vi "Day 3 DataFlow Tasks.vi"() -> ()   [LabVIEW 2026]
panel:
  out "Final Result 7":dbl
  in  "D1 3":dbl
  in  "C1 3":dbl
  in  "B1 3":dbl
  in  "A1 3":dbl
  out "Division Result 6":dbl
  in  "M 3":dbl
  in  "L 3":dbl
  out "Final Result 6":dbl
  in  "D1 2":dbl
  in  "C1 2":dbl
  in  "B1 2":dbl
  in  "A1 2":dbl
  out "Division Result 5":dbl
  in  "M 2":dbl
  in  "L 2":dbl
  out "Final Result 5":dbl
  in  "D1":dbl
  in  "C1":dbl
  in  "B1":dbl
  in  "A1":dbl
  out "Division Result 4":dbl
  in  "M":dbl
  in  "L":dbl
  in  "P 2":dbl
  in  "Q 2":dbl
  in  "R 2":dbl
  in  "S 2":dbl
  out "Final Result 4":dbl
  in  "X 3":dbl
  in  "Y 3":dbl
  out "Division Result 3":dbl
  out "Final Result 3":dbl
  in  "S":dbl
  in  "R":dbl
  in  "Q":dbl
  in  "P":dbl
  out "Division Result 2":dbl
  in  "Y 2":dbl
  in  "X 2":dbl
  out "Final Result 2":dbl
  in  "D 2":dbl
  in  "C 2":dbl
  in  "B 2":dbl
  in  "A 2":dbl
  out "Division Result":dbl
  in  "Y":dbl
  in  "X":dbl
  out "Final Result":dbl
  in  "D":dbl
  in  "C":dbl
  in  "B":dbl
  in  "A":dbl
  # "Task 1 : Wire a chain of arithmetic primitives and predict the execution order from dataflow."
  # "Task 3 :  Take a VI written with a Sequence structure and rewrite it to rely on  dataflow alone."
  # "Task 2 : Build a VI with two independent branches; explain which executes first and why."
  # "Trying the above system to make it entirely rely on DataFlow without Flat Sequence VERSION LAST but it chnages the math Value"
  # "Trying the above system to make it entirely rely on DataFlow without Flat Sequence VERSION 1"
  # "Trying the above system to make it entirely rely on DataFlow without Flat Sequence \n                                           VERSION 4 SELECTOR FUNCTION"
  # "Trying the above system to make it entirely rely on DataFlow without Flat Sequence VERSION 3"
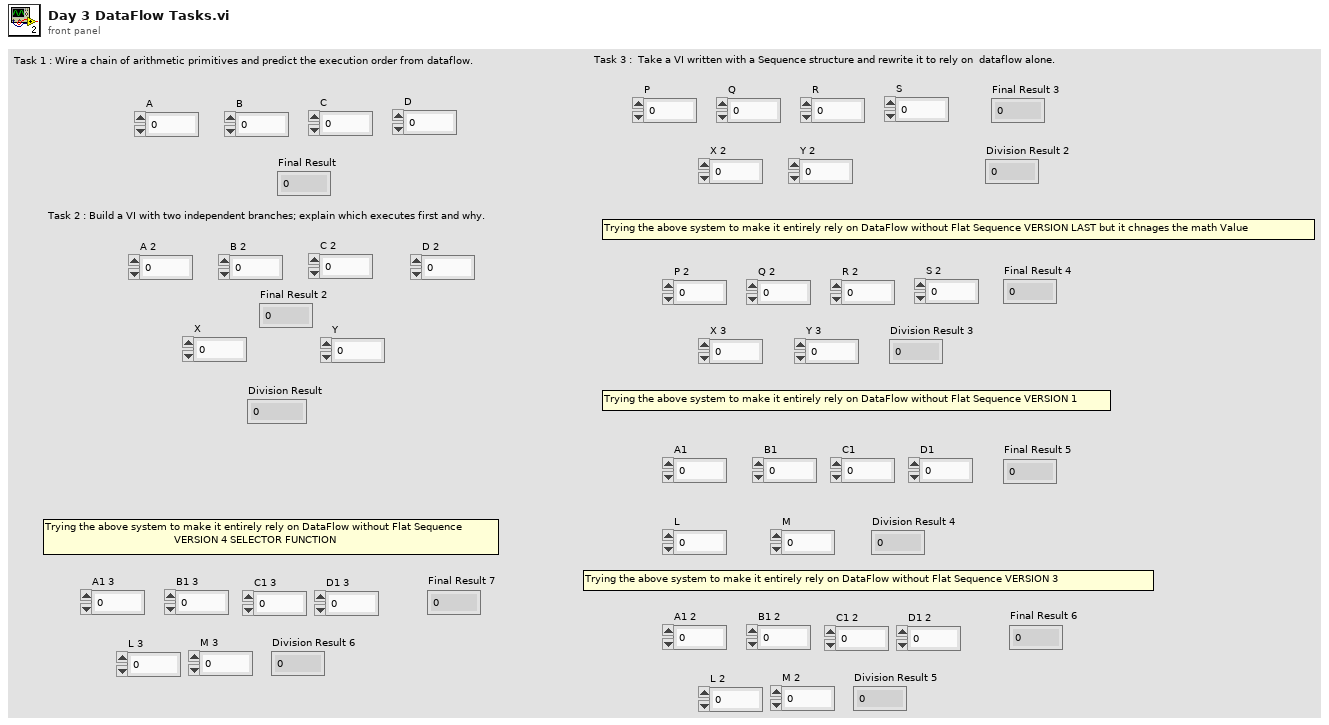
[diagram p1: front panel]
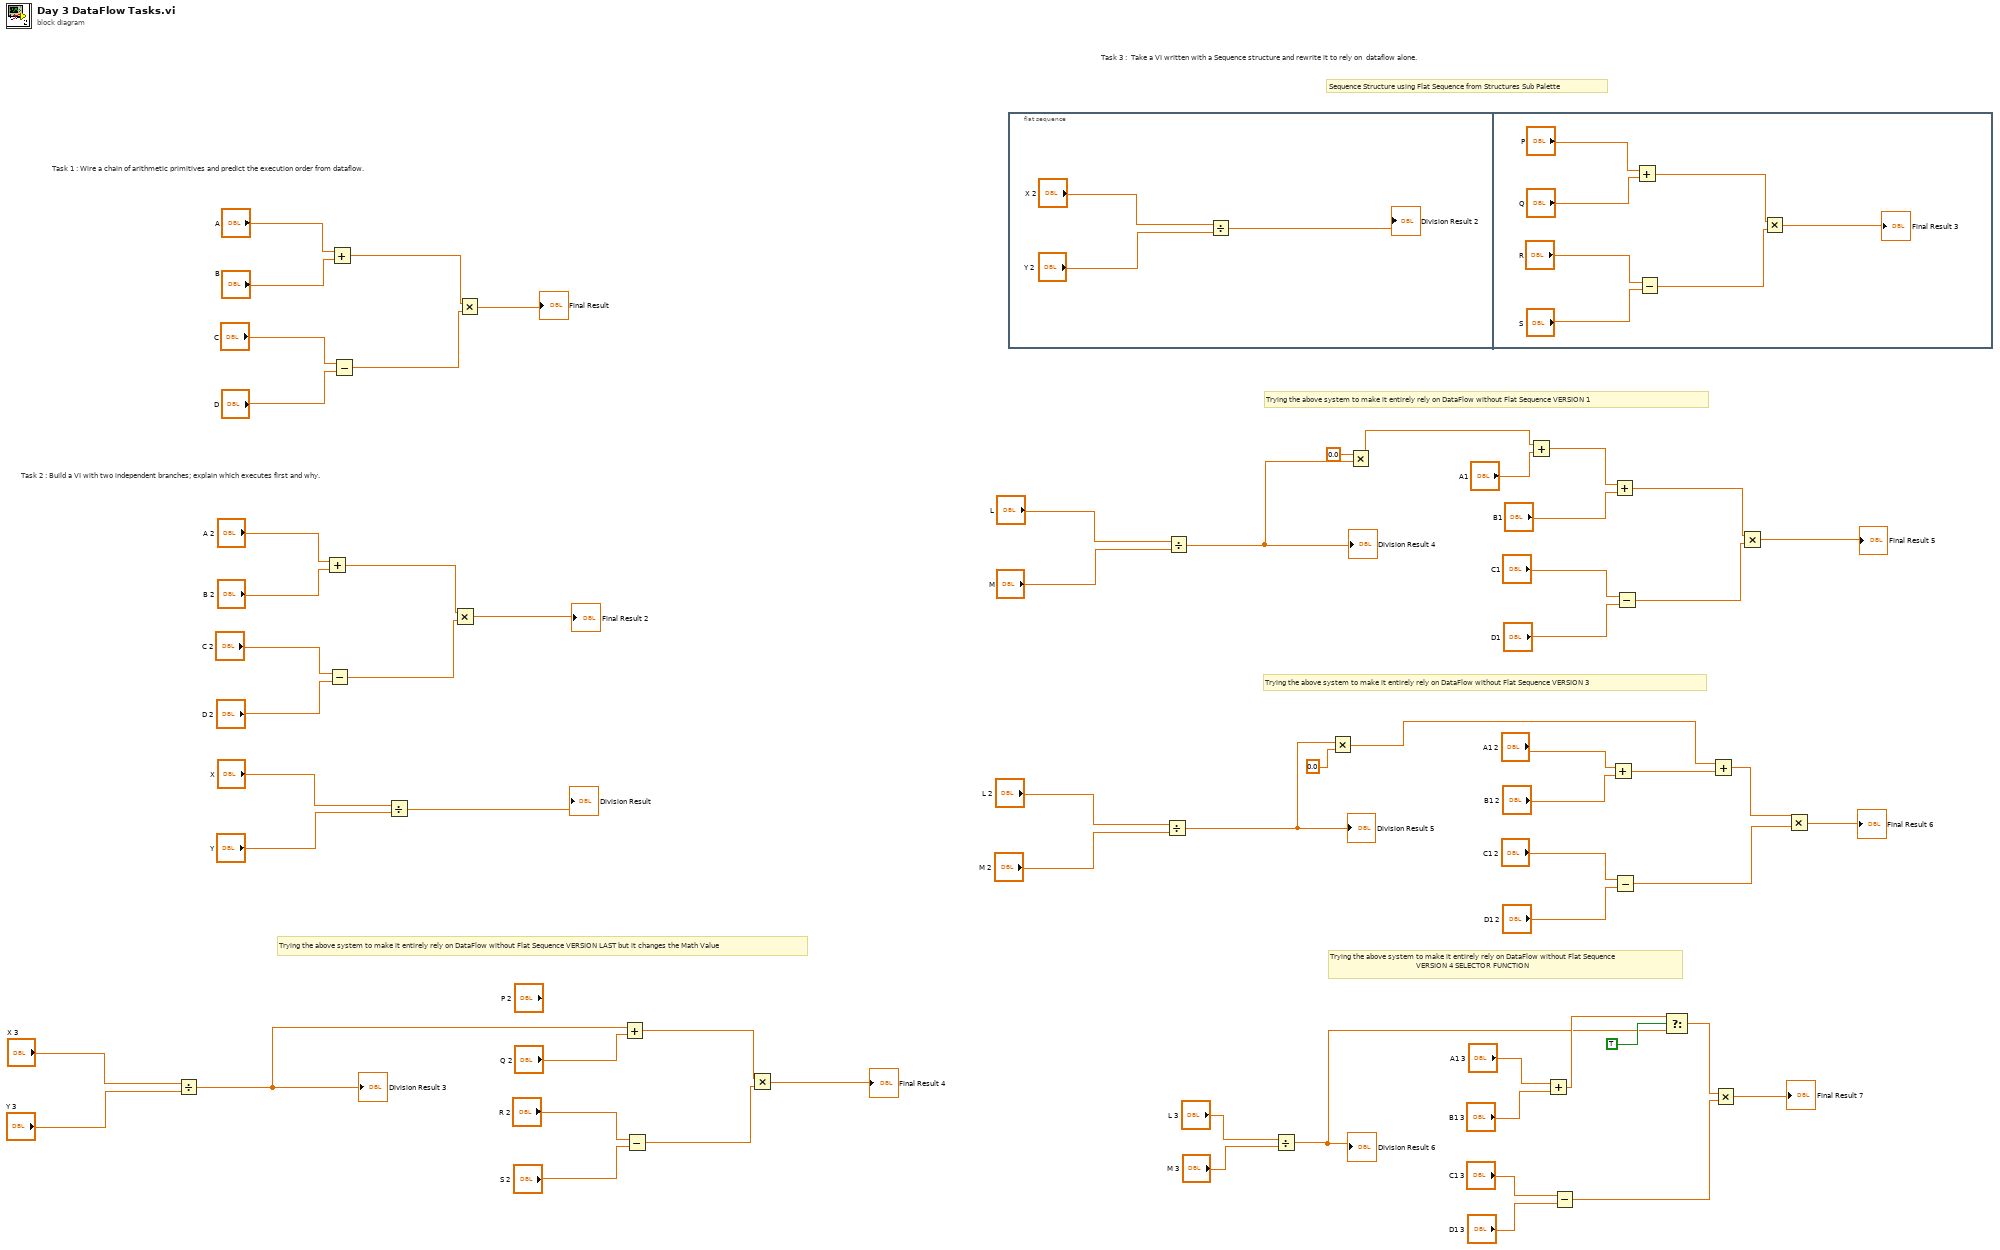
[diagram p0: block diagram]
diagram:
  # "Trying the above system to make it entirely rely on DataFlow without Flat Sequence \n                                           VERSION 4 SELECTOR FUNCTION"
  # "Trying the above system to make it entirely rely on DataFlow without Flat Sequence VERSION 3"
  # "Trying the above system to make it entirely rely on DataFlow without Flat Sequence VERSION 1"
  # "Trying the above system to make it entirely rely on DataFlow without Flat Sequence VERSION LAST but it changes the Math Value"
  # "Sequence Structure using Flat Sequence from Structures Sub Palette"
  # "Task 3 :  Take a VI written with a Sequence structure and rewrite it to rely on  dataflow alone."
  # "Task 2 : Build a VI with two independent branches; explain which executes first and why."
  # "Task 1 : Wire a chain of arithmetic primitives and predict the execution order from dataflow."
  n1 = Divide(x="X 3", y="Y 3") -> (x/y=w39:dbl)
  "Division Result 3" <- w39
  n2 = Add(x="A 2", y="B 2") -> (x+y=w48:dbl)
  n3 = Subtract(x="C 2", y="D 2") -> (x-y=w51:dbl)
  n4 = Add(x="A", y="B") -> (x+y=w58:dbl)
  n5 = Subtract(x="C", y="D") -> (x-y=w61:dbl)
  n6 = Divide(x="X", y="Y") -> (x/y=→"Division Result":dbl)
  n7 = Multiply(x=w48, y=w51) -> (x*y=→"Final Result 2":dbl)
  n8 = Multiply(x=w58, y=w61) -> (x*y=→"Final Result":dbl)
  n9 = Add(x=w39, y="Q 2") -> (x+y=w45:dbl)
  n10 = Subtract(x="R 2", y="S 2") -> (x-y=w43:dbl)
  n11 = Multiply(x=w45, y=w43) -> (x*y=→"Final Result 4":dbl)
  n12 = flat-sequence {
    frame #0 {
      n13 = Divide(x="X 2", y="Y 2") -> (x/y=→"Division Result 2":dbl)
    }
    frame #1 {
      n14 = Add(x="P", y="Q") -> (x+y=w74:dbl)
      n15 = Subtract(x="R", y="S") -> (x-y=w71:dbl)
      n16 = Multiply(x=w74, y=w71) -> (x*y=→"Final Result 3":dbl)
    }
  }
  n17 = Divide(x="L 2", y="M 2") -> (x/y=w17:dbl)
  "Division Result 5" <- w17
  n18 = Divide(x="L", y="M") -> (x/y=w28:dbl)
  "Division Result 4" <- w28
  n19 = Divide(x="L 3", y="M 3") -> (x/y=w1:dbl)
  "Division Result 6" <- w1
  n20 = Multiply(x=w17, y=0.0) -> (x*y=w15:dbl)
  n21 = Multiply(x=0.0, y=w28) -> (x*y=w26:dbl)
  n22 = Add(x=w26, y="A1") -> (x+y=w29:dbl)
  n23 = Add(x="A1 3", y="B1 3") -> (x+y=w2:dbl)
  n24 = Subtract(x="C1 3", y="D1 3") -> (x-y=w6:dbl)
  n25 = Add(x="A1 2", y="B1 2") -> (x+y=w14:dbl)
  n26 = Add(x=w29, y="B1") -> (x+y=w36:dbl)
  n27 = Subtract(x="C1 2", y="D1 2") -> (x-y=w22:dbl)
  n28 = Subtract(x="C1", y="D1") -> (x-y=w34:dbl)
  n29 = Select(t=w2, s=TRUE, f=w1) -> (s? t:f=w3:dbl)
  n30 = Add(x=w15, y=w14) -> (x+y=w13:dbl)
  n31 = Multiply(x=w3, y=w6) -> (x*y=→"Final Result 7":dbl)
  n32 = Multiply(x=w36, y=w34) -> (x*y=→"Final Result 5":dbl)
  n33 = Multiply(x=w13, y=w22) -> (x*y=→"Final Result 6":dbl)
